vi "Debug LV API.vi"() -> ()   [LabVIEW 2023]
doc: "Example to verify functionality using LV Host APIs"
panel:
  in  "Output channel name":string[](array[string])=["Connector0_DIOPORT2", "Connector0_DIOPORT3", "Connector1_DIOPORT2", "Connector1_DIOPORT3"]
  in  "Channel data":u8[](array[numeric])=[255, 50, 100, 200]
  in  "Input channel names":string[](array[string])=["Connector0_DIOPORT0", "Connector0_DIOPORT1", "Connector1_DIOPORT0", "Connector1_DIOPORT1"]
  in  "Bit file path":path
  in  "Resource":string="Digital_RIO_7822R"
  out "error out":errorcluster
  out "Channel data out":u8[](array[numeric])
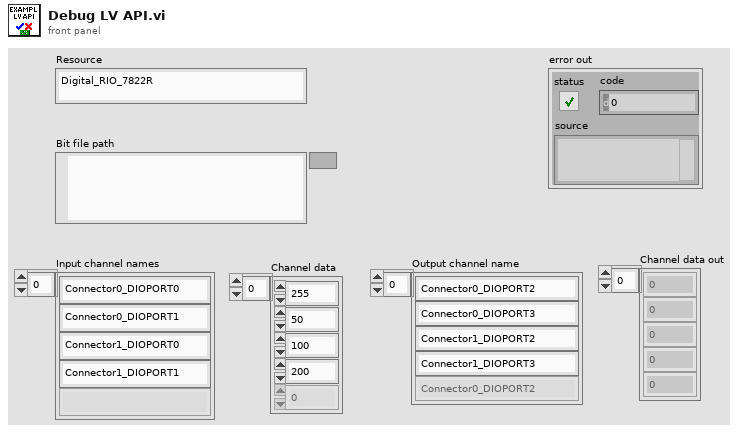
[diagram p1: front panel]
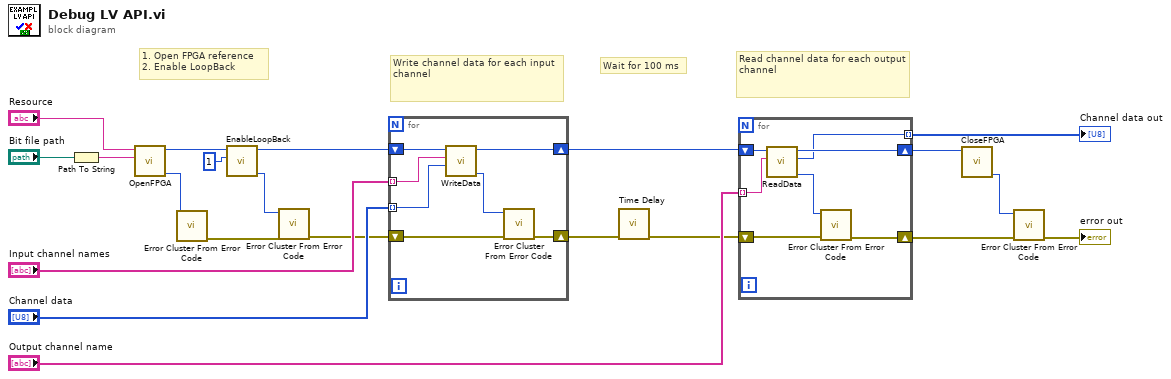
[diagram p0: block diagram]
diagram:
  # "Read channel data for each output channel"
  # "Wait for 100 ms"
  # "Write channel data for each input channel"
  # "1. Open FPGA reference\n2. Enable LoopBack"
  n1 = Path To String(path="Bit file path") -> (string=w15:string)
  n2 = call "OpenFPGA.vi"("FPGA bit file path"=w15, "Resource name"="Resource") -> ("Error code"=w9:i32, "Reference ID"=w14:u64)  [unwired: 8 in]
  n3 = call <vilib>:"Error Cluster From Error Code.vi"("error code (0)"=w9) -> ("error out"=w7:errorcluster)  [unwired: 8 in]
  n4 = call "EnableLoopBack.vi"("Enable Loopback"=u64 1, "Reference ID"=w14) -> ("Error code"=w8:i32, "Reference ID out"=w12:u64)  [unwired: 8 in]
  n5 = call <vilib>:"Error Cluster From Error Code.vi"("error in (no error)"=w7, "error code (0)"=w8) -> ("error out"=w6:errorcluster)  [unwired: 7 in]
  n6 = for {
    tunnel: "Input channel names" -> [w26] mode=indexing
    tunnel: "Channel data" -> [w27] mode=indexing
    shift-right: [w25] -> w11
    shift-left: w12 -> [w28]
    shift-right: [w22] -> w2
    shift-left: w6 -> [w23]
    n7 = call "WriteData.vi"("Channel Data"=w27, "Channel name"=w26, "Reference ID"=w28) -> ("Error code"=w24:i32, "Reference ID out"=w25:u64)  [unwired: 7 in]
    n8 = call <vilib>:"Error Cluster From Error Code.vi"("error in (no error)"=w23, "error code (0)"=w24) -> ("error out"=w22:errorcluster)  [unwired: 7 in]
  }
  n9 = call "Time Delay"("error in (no error)"=w2) -> ("error out"=w1:errorcluster)  [unwired: 10 in]
  n10 = for {
    tunnel: "Output channel name" -> [w34] mode=indexing
    tunnel: [w32] -> w19 mode=indexing
    shift-right: [w33] -> w10
    shift-left: w11 -> [w35]
    shift-right: [w29] -> w4
    shift-left: w1 -> [w31]
    n11 = call "ReadData.vi"("Channel name"=w34, "Reference ID"=w35) -> ("Error code"=w30:i32, "Channel data"=w32:u8, "Reference ID out"=w33:u64)  [unwired: 7 in]
    n12 = call <vilib>:"Error Cluster From Error Code.vi"("error in (no error)"=w31, "error code (0)"=w30) -> ("error out"=w29:errorcluster)  [unwired: 7 in]
  }
  "Channel data out" <- w19
  n13 = call "CloseFPGA.vi"("Reference ID"=w10) -> ("Error code"=w5:i32)  [unwired: 10 in]
  n14 = call <vilib>:"Error Cluster From Error Code.vi"("error in (no error)"=w4, "error code (0)"=w5) -> ("error out"=→"error out":errorcluster)  [unwired: 7 in]
